vi "PoC.vi"() -> ()   [LabVIEW 2021]
uses:
  <vilib>/Utility/file.llb/Read Delimited Spreadsheet (string).vi
panel:
  out "Table":string[][](table)
  in  "file path (dialog if empty)":path
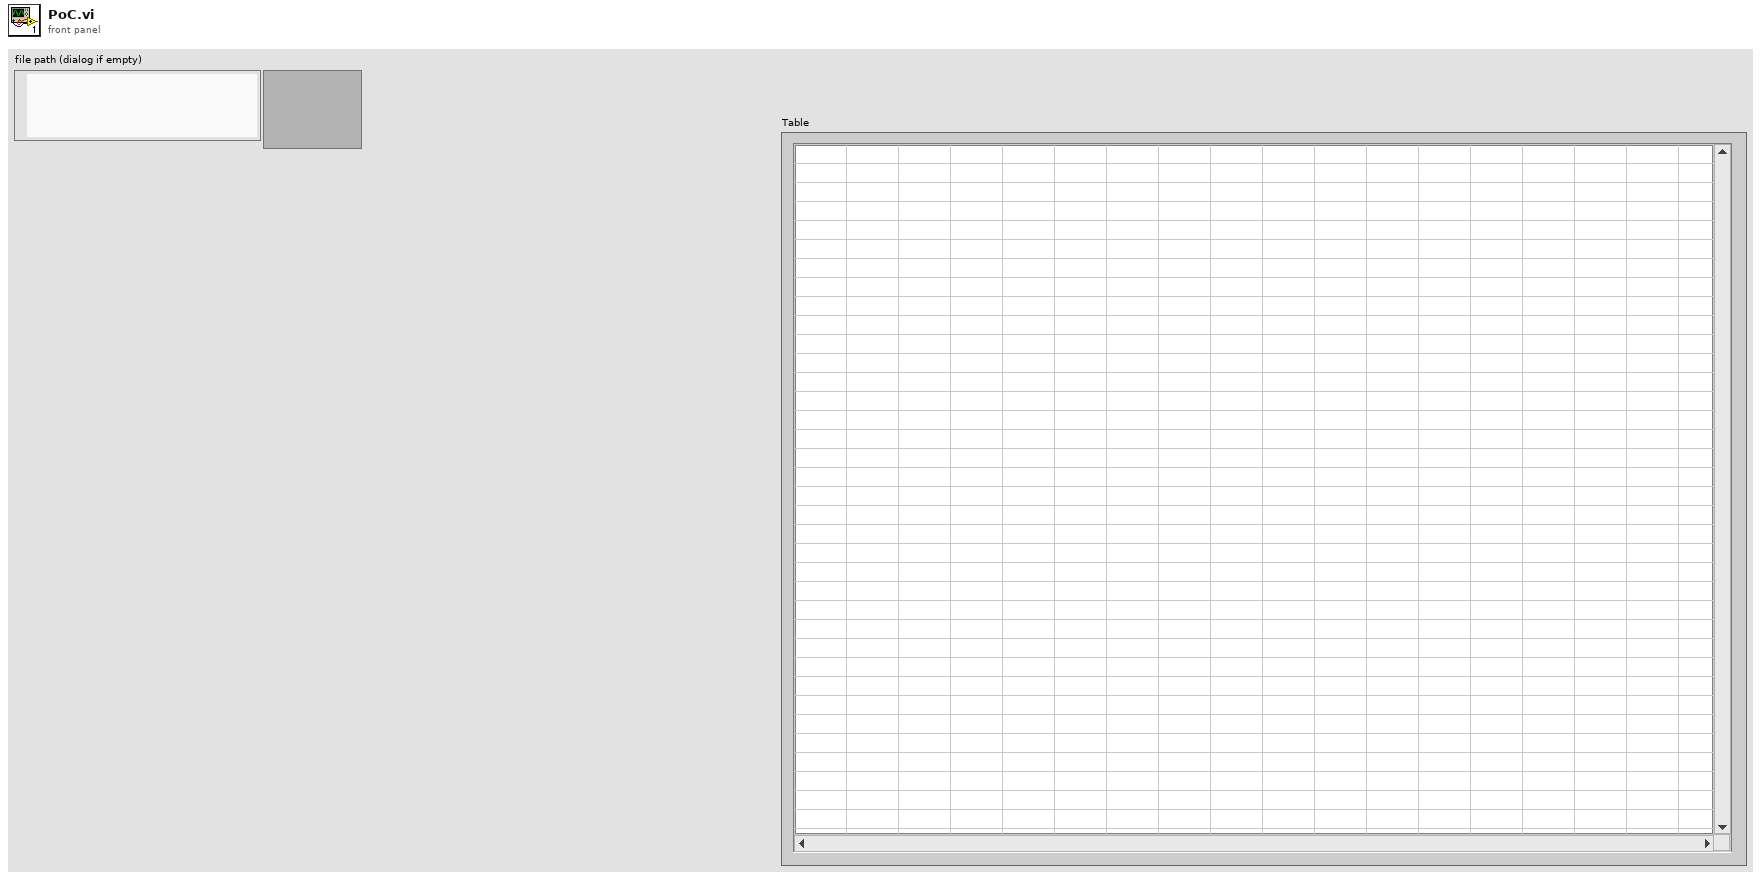
[diagram p1: front panel]
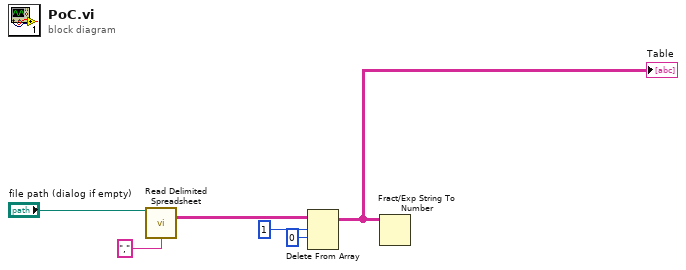
[diagram p0: block diagram]
diagram:
  n1 = call-poly <vilib>:"Read Delimited Spreadsheet.vi"("file path (dialog if empty)"="file path (dialog if empty)", "delimiter (\\t)"="," ("delimiter (\\t)")) -> ("all rows"=w4:string[][])  [unwired: 8 in, 5 out]
  n2 = Delete From Array(array=w4, length=1, index (row)=0) -> (array with subset deleted=w1:string[][])  [unwired: 1 in, 1 out]
  "Table" <- w1
  n3 = Fract/Exp String To Number(string=w1) -> ()  [unwired: 3 in, 2 out]
